vi "未命名 2.vi"() -> ()   [LabVIEW 2021]
uses:
  scoure/WebFaceAPI/BaiduFaceAPI.lvlib
panel:
  in  "人脸参数":T1={"max_face_num"=32, "face_fields 2"={"age"=FALSE, "beauty"=FALSE, "expression"=FALSE, "faceshape"=FALSE, "gender"=FALSE, "glasses"=FALSE, "landmark"=FALSE, "race"=FALSE, "qualities"=FALSE}, "image"=""}
  out "body":string caption="体部"
  in  "路径":path
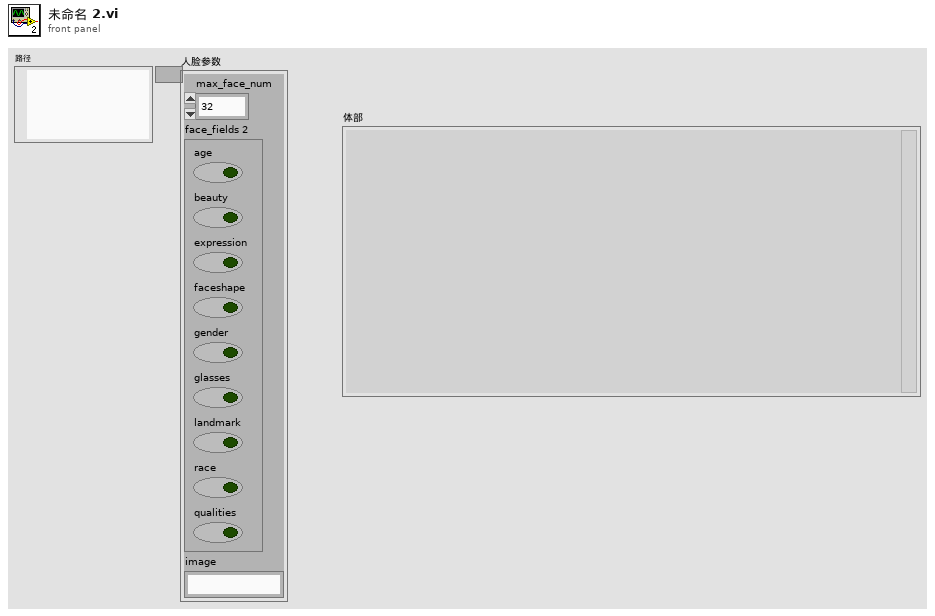
[diagram p1: front panel]
types:
  T1 = cluster{"max_face_num":u32, "face_fields 2":cluster{"age":bool, "beauty":bool, "expression":bool, "faceshape":bool, "gender":bool, "glasses":bool, "landmark":bool, "race":bool, "qualities":bool}, "image":string}
  T2 = typedef "Image Type" = u32
  T3 = typedef "IMAQ Image.ctl" = refnum<image>
  T4 = typedef "LabVIEWHTTPClient.lvlib/ClientHandle.ctl" = refnum<k1>
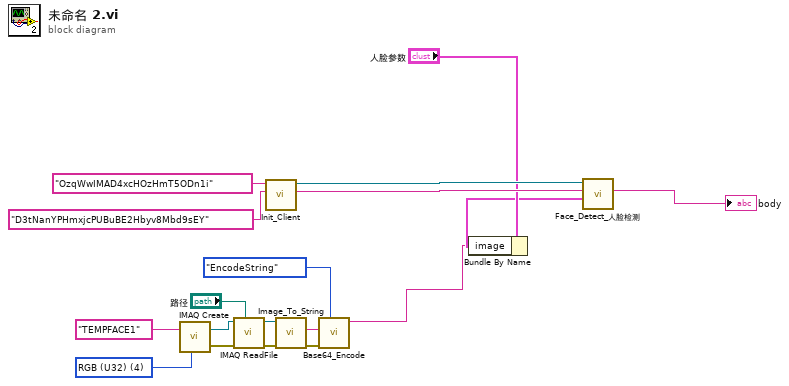
[diagram p0: block diagram]
diagram:
  w12 = T2 4 items=["Grayscale (U8)", "Grayscale (I16)", "Grayscale (SGL)", "Complex (CSG)", "RGB (U32)", "HSL (U32)", "RGB (U64)", "Grayscale (U16)"] ("Image Type")
  n1 = call "IMAQ Create"("Image Name"="TEMPFACE1", "Image Type"=w12) -> ("New Image"=w6:T3, "error out"=w4:errorcluster)  [unwired: 3 in]
  n2 = call "IMAQ ReadFile"("File Path"="路径", "error in (no error)"=w4, "Image"=w6) -> ("error out"=w3:errorcluster, "Image Out"=w7:T3)  [unwired: 4 in, 3 out]
  n3 = call "Init_Client.vi"("Secret Key"="D3tNanYPHmxjcPUBuBE2Hbyv8Mbd9sEY", "API Key"="OzqWwIMAD4xcHOzHmT5ODn1i") -> ("access_token"=w15:string, "client_out"=w16:T4)  [unwired: 7 in, 1 out]
  n4 = call "Image_To_String.vi"("错误输入（无错误）"=w3, "引用句柄输入"=w7) -> ("错误输出"=w10:errorcluster, "FileString"=w9:string)  [unwired: 7 in, 1 out]
  n5 = call "Base64_Encode.vi"("枚举"=enum16{"EncodeString", "EcodeFile"}."EncodeString", "错误输入"=w10, "字符串"=w9) -> ("encodeURIComponent"=w1:string)  [unwired: 5 in, 3 out]
  n6 = Bundle By Name(cluster="人脸参数", "image"=w1) -> (w13:T1)
  n7 = call "Face_Detect_人脸检测.vi"("人脸参数"=w13, "access_token"=w15, "client_in"=w16) -> ("body"=→"body":string)  [unwired: 6 in, 2 out]
